vi "slopes2command_test.vi"() -> ()   [LabVIEW 2018]
uses:
  <userlib>/WaveKit.lib/Controls/HasoSlopes.lvclass
  <userlib>/WaveKit.lib/Classes/CorrectionDataManager/CorrectionDataManager.lvclass
  <userlib>/WaveKit.lib/Controls/InteractionMatrixToCommandMatrixParameters.ctl
panel:
  in  "Hasao configuration file":path=path "D:/YD/data/20191206/im.aomi"
  in  "interaction matrix file":path=path "D:/YD/data/20191206/im.aomi"
  in  "Initial haso file":path=path "D:/SystemAlignment/system_aberration_20191029.dat"
  out "Offset Positions":sgl[](array[numeric])
  in  "Output folder":path=path "D:/Data/20200122_Test"
  in  "Output file name":string="Data\\data_image.himg"
  out "error out":errorcluster
  in  "error in (no error)":errorcluster
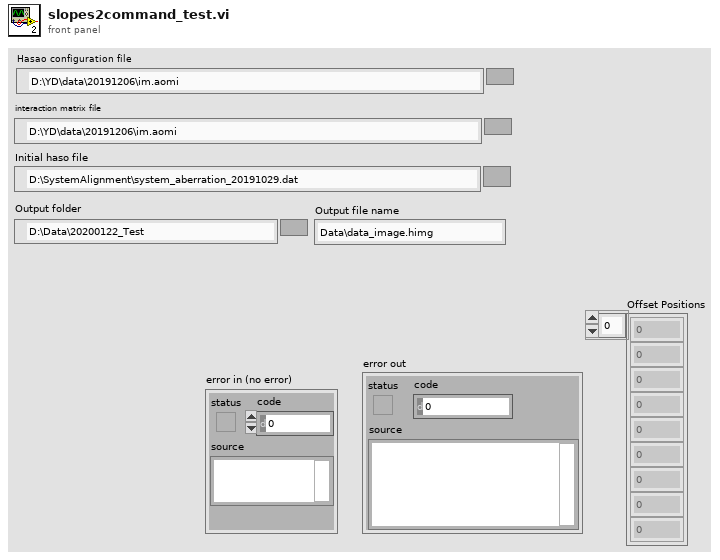
[diagram p1: front panel]
types:
  T1 = typedef "InteractionMatrixToCommandMatrixParameters.ctl" = cluster{"Number of kept modes":i32, "Tilt filtering":bool}
  T2 = typedef "Wavefront Corrector Position.ctl" = sgl[]
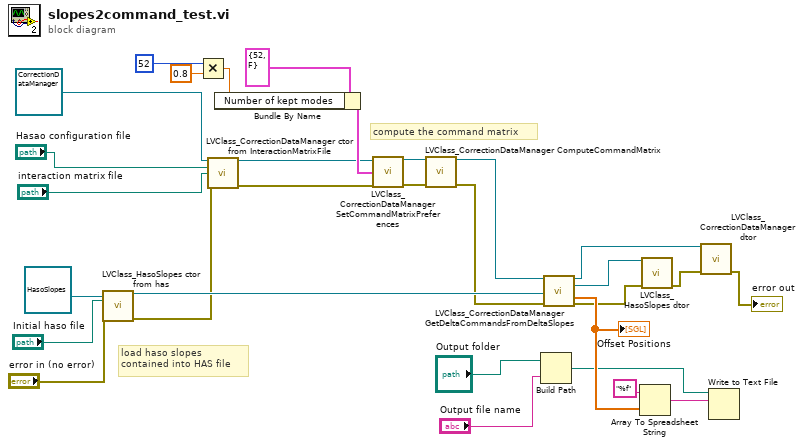
[diagram p0: block diagram]
diagram:
  # "compute the command matrix"
  # "load haso slopes\ncontained into HAS file"
  n1 = call <userlib>:"LVClass_HasoSlopes ctor from has.vi"("HasoSlopes in"=refnum<class "HasoSlopes.lvclass"> refnum, ".has path"="Initial haso file", "error in (no error)"="error in (no error)") -> ("HasoSlopes out"=w21:refnum<class "HasoSlopes.lvclass">, "error out"=w18:errorcluster)  [unwired: 11 in]
  n2 = Multiply(x=52 ("Number of kept modes"), y=0.8) -> (x*y=w14:dbl)
  n3 = call <userlib>:"LVClass_CorrectionDataManager ctor from InteractionMatrixFile.vi"("CorrectionDataManager in"=refnum<class "CorrectionDataManager.lvclass"> refnum, "Haso config file path"="Hasao configuration file", "Interaction matrix path"="interaction matrix file", "error in (no error)"=w18) -> ("CorrectionDataManager out"=w10:refnum<class "CorrectionDataManager.lvclass">, "error out"=w9:errorcluster)  [unwired: 10 in]
  n4 = Bundle By Name(cluster=T1 {"Number of kept modes"=52, "Tilt filtering"=FALSE} ("Prefs"), "Number of kept modes"=w14) -> (w13:T1)
  n5 = call <userlib>:"LVClass_CorrectionDataManager SetCommandMatrixPreferences.vi"("CorrectionDataManager in"=w10, "Prefs"=w13, "error in (no error)"=w9) -> ("CorrectionDataManager out"=w17:refnum<class "CorrectionDataManager.lvclass">, "error out"=w12:errorcluster)  [unwired: 11 in]
  n6 = call <userlib>:"LVClass_CorrectionDataManager ComputeCommandMatrix.vi"("CorrectionDataManager in"=w17, "error in (no error)"=w12) -> ("CorrectionDataManager out"=w8:refnum<class "CorrectionDataManager.lvclass">, "error out"=w7:errorcluster)  [unwired: 12 in]
  n7 = Build Path(base path="Output folder", name or relative path="Output file name") -> (appended path=w25:path)
  n8 = call <userlib>:"LVClass_CorrectionDataManager GetDeltaCommandsFromDeltaSlopes.vi"("CorrectionDataManager in"=w8, "Delta Slopes IN"=w21, "error in (no error)"=w7) -> ("CorrectionDataManager out"=w6:refnum<class "CorrectionDataManager.lvclass">, "Delta Slope OUT"=w5:refnum<class "HasoSlopes.lvclass">, "DeltaPosition"=w28:T2, "error out"=w4:errorcluster)  [unwired: 8 in, 1 out]
  "Offset Positions" <- w28
  n9 = Array To Spreadsheet String(array=w28, 3:"%f") -> (spreadsheet string=w29:string)  [unwired: 1 in]
  n10 = call <userlib>:"LVClass_HasoSlopes dtor.vi"("HasoSlopes in"=w5, "error in (no error)"=w4) -> ("error out"=w3:errorcluster)  [unwired: 12 in, 1 out]
  n11 = call <userlib>:"LVClass_CorrectionDataManager dtor.vi"("CorrectionDataManager in"=w6, "error in (no error)"=w3) -> ("error out"=→"error out":errorcluster)  [unwired: 12 in, 1 out]
  n12 = Write to Text File(file (use dialog)=w25, text=w29) -> ()  [unwired: 2 in, 3 out]
